vi "Set Waveform Label.vi"(8 "error in (no error)":errorcluster, 9 "Label":string, 10 "Analog Channels":T1, 11 "PicoScope 3000a in":refnum<class "PicoScope 3000a.lvclass">) -> (0 "error out":errorcluster, 3 "PicoScope 3000a out":refnum<class "PicoScope 3000a.lvclass">)   [LabVIEW 2018, in "PicoScope 3000a.lvlib" / "PicoScope 3000a.lvclass"]
doc: "This Override is used to label channel waveforms."
uses:
  PicoScope 3000a.lvclass
  PPLs/Oscilloscope/Parent/Oscilloscope.lvlibp/Custom Controls/Analog Channels.ctl
  PPLs/Oscilloscope/Parent/Oscilloscope.lvlibp
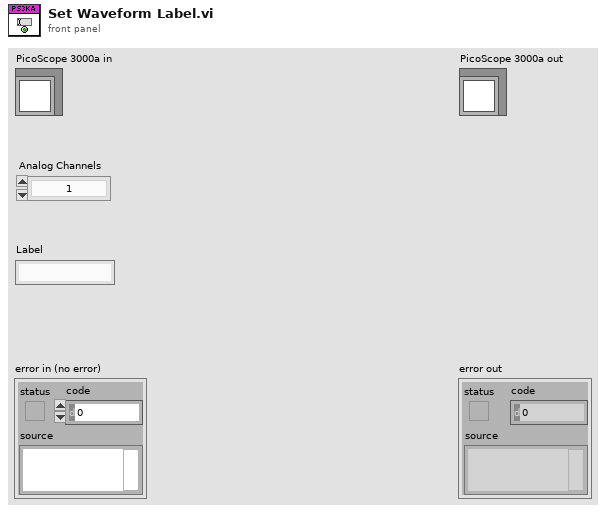
[diagram p1: front panel]
types:
  T1 = typedef "Oscilloscope.lvlibp/Analog Channels.ctl" = enum16{"1", "2", "3", "4", "5", "6", "7", "8", "9", "10", "11", "12", "13", "14", "15", "16"}
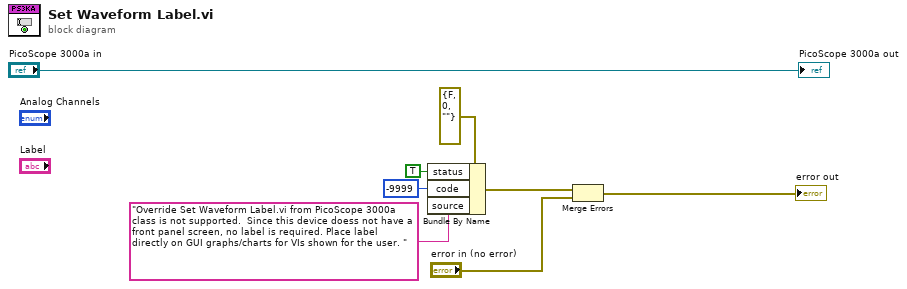
[diagram p0: block diagram]
diagram:
  n1 = Bundle By Name(cluster=errorcluster {"status"=FALSE, "code"=0, "source"=""} ("error constant"), "status"=TRUE, "code"=-9999, "source"="Override Set Waveform Label.vi from PicoScope 3000a class is not supported.  Since this device doess not have a front panel screen, no label is required. Place label directly on GUI graphs/charts for VIs shown for the user. ") -> (w4:errorcluster)
  n2 = Merge Errors(w4, "error in (no error)") -> (→"error out":errorcluster)
  "PicoScope 3000a out" <- "PicoScope 3000a in"
